vi "Drive For Time Robot Centric.vi"(0 "Left/right":dbl, 1 "Forward/Backwards":dbl, 3 "Rotation":dbl, 4 "Seconds":dbl, 5 "Command Info In":T1, 6 "Description":string, 7 "Synchronization":enum16{"Start", "Wait"}(ring), 10 "Collsision Detection":bool, 11 "POV":i16, 15 "Tracks":bool) -> (14 "Outcome":string="foo", 19 "Command Info Out":T1)   [LabVIEW 2017]
doc: "This VI sets the motors to run for a given number of seconds. It optionally synchronizes with the completion of the command."
uses:
  <vilib>/Rock Robotics/WPI/Framework/Command Status Info.ctl
  <vilib>/Rock Robotics/WPI/Framework/Completion Status.ctl
  <vilib>/Rock Robotics/WPI/Framework/Completion Notifier.ctl
  Implementation/Drive Setpoints.ctl
  Implementation/Drive Operations.ctl
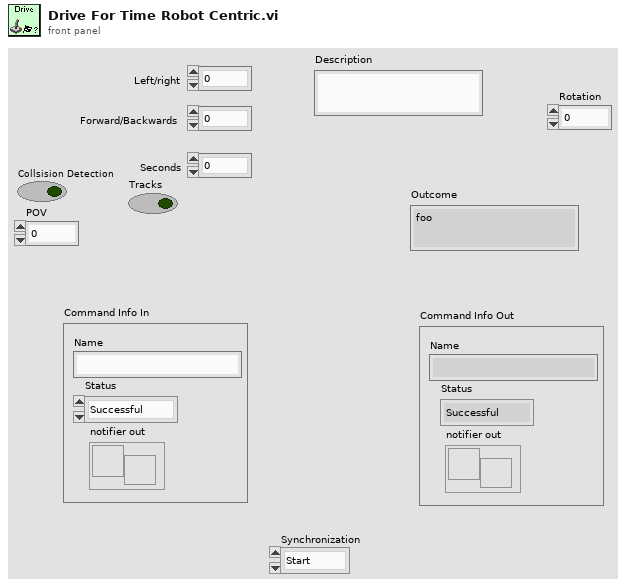
[diagram p1: front panel]
types:
  T1 = typedef "Command Status Info.ctl" = cluster{"Name":string, "Status":T2, "notifier out":T3}
  T2 = typedef "Completion Status.ctl" = enum16{"Successful", "Aborted", "Incomplete"}
  T3 = typedef "Completion Notifier.ctl" = refnum<notifier>
  T4 = typedef "Drive Setpoints.ctl" = cluster{"Operation":T5, "X Setpoint":dbl, "Y Setpoint":dbl, "Duration":dbl, "Z Setpoint":dbl, "Tracks":bool, "Gyro":dbl, "POV":i16, "Distance(feet)":dbl, "AutoTrack Toggle":bool, "Collsision Detection":bool, "Reset Encoder":bool, "MP File Name":string}
  T5 = typedef "Drive Operations.ctl" = enum16{"Reserve", "Read Current", "Reset Motors VBus", "Motion Profile run", "Motion Profiling Get Time", "Immediate Robot Centric", "Drive for Time Robot Centric", "Immediate Field Centric", "Drive For Time Field Centric", "Immediate MecaTrak", "Push Motion Profile", "Drive For Time MecaTrak", "Button Adjust", "Drive for Distance", "Drive Directional Immediate"}
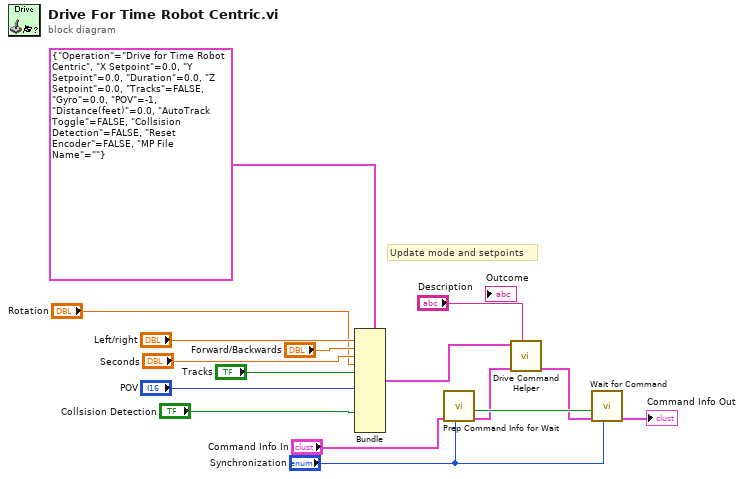
[diagram p0: block diagram]
diagram:
  # "Update mode and setpoints"
  n1 = Bundle(cluster=T4 {"Operation"=enum."Drive for Time Robot Centric", "X Setpoint"=0.0, "Y Setpoint"=0.0, "Duration"=0.0, "Z Setpoint"=0.0, "Tracks"=FALSE, "Gyro"=0.0, "POV"=-1, "Distance(feet)"=0.0, "AutoTrack Toggle"=FALSE, "Collsision Detection"=FALSE, "Reset Encoder"=FALSE, "MP File Name"=""} ("SubSystem Data"), "X Setpoint"="Left/right", "Y Setpoint"="Forward/Backwards", "Duration"="Seconds", "Z Setpoint"="Rotation", "Tracks"="Tracks", "Distance(feet)"="POV", "Collsision Detection"="Collsision Detection") -> (w8:T4)  [unwired: 6 in]
  n2 = call <vilib>:"Prep Command Info for Wait.vi"("Synchronication"="Synchronization", "Command Info"="Command Info In") -> ("Command Info"=w12:T1, "Allocated"=w13:bool)  [unwired: 8 in]
  n3 = call "Drive Command Helper.vi"("Description"="Description", "Command Info In"=w12, "SubSystem Data"=w8) -> ("Command Info Out"=w9:T1)  [unwired: 7 in, 1 out]
  n4 = call <vilib>:"Wait for Command.vi"("Synchronication"="Synchronization", "Command Info in"=w9, "Allocated"=w13) -> ("Command Info out"=→"Command Info Out":T1)  [unwired: 8 in]
